vi "Cuenta.vi"(8 "error in (no error)":errorcluster, 11 "Contador Binario in":refnum<class "Contador Binario.lvclass">) -> (0 "error out":errorcluster, 3 "Contador Binario out":refnum<class "Contador Binario.lvclass">)   [LabVIEW 2020, in "Contador Binario.lvlib" / "Contador Binario.lvclass"]
uses:
  Contador Binario.lvclass
  Contador Binario.lvclass/Contador Binario.ctl
  Logging Txt/Logging Txt Messages/Save data Msg/Save data Msg.lvclass/Save data Msg.ctl
  <vilib>/ActorFramework/Message Enqueuer/Message Enqueuer.lvclass/Message Enqueuer.ctl
  <vilib>/ActorFramework/Message Enqueuer/Enqueue.vi
  Logging Txt/Logging Txt Messages/Save data Msg/Save data Msg.lvclass
  C:/Program Files (x86)/National Instruments/LabVIEW 2020/vi.lib/ActorFramework/Message/Message.lvclass
  <vilib>/ActorFramework/Message Priority Queue/Priority Enqueue.vi
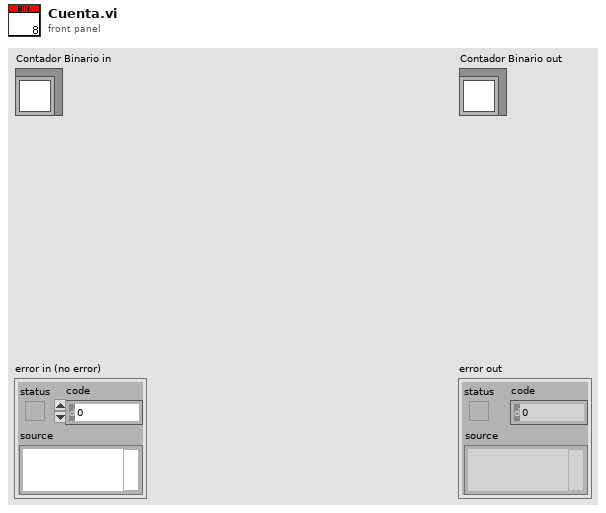
[diagram p1: front panel]
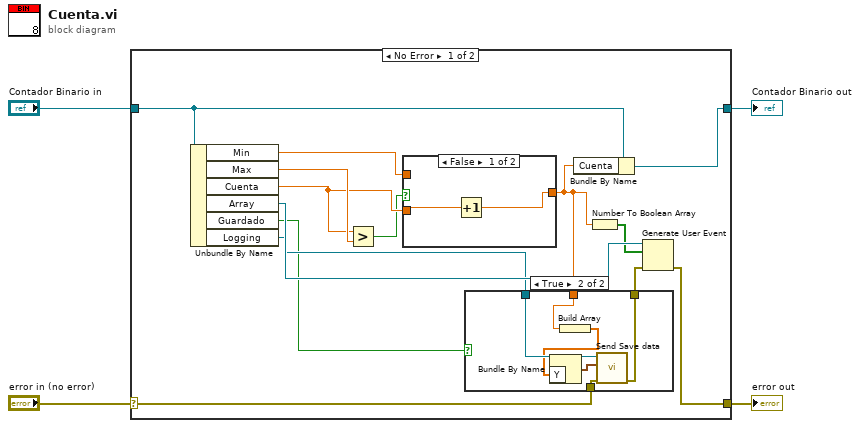
[diagram p0: block diagram]
diagram:
  n1 = case shown="No Error" "error in (no error)" {
    selector: "error in (no error)" -> [w7 w30]
    tunnel: [w5 w30] -> w3
    tunnel: [w17 w29] -> w1
    tunnel: "Contador Binario in" -> [w18 w29]
    frame No Error {
      n2 = Unbundle By Name(w18) -> ("Min"=w14:dbl, "Max"=w16:dbl, "Cuenta"=w15:dbl, "Array"=w12:refnum<user-event>, "Guardado"=w9:bool, "Logging"=w10:refnum<class "Message Enqueuer.lvclass">)
      n3 = Greater?(x=w15, y=w16) -> (0:w13:bool)
      n4 = case shown="False" w13 {
        tunnel: w15 -> [w26 _]
        tunnel: [w27 w28] -> w8
        tunnel: w14 -> [_ w28]
        frame False {
          n5 = Increment(x=w26) -> (x+1=w27:dbl)
        }
        frame True {
        }
      }
      n6 = case shown="True" w9 {
        tunnel: w10 -> [_ w25]
        tunnel: w8 -> [_ w23]
        tunnel: w7 -> [w19 w21]
        tunnel: [w19 w20] -> w6
        frame False {
        }
        frame True {
          n7 = Build Array(w23) -> (w22:dbl[])
          n8 = Bundle By Name("Y"=w22) -> (w24:waveform(dbl))  [unwired: 1 in]
          n9 = call "Send Save data.vi"("error in (no error)"=w21, "signal out"=w24, "Message Enqueuer"=w25) -> ("error out"=w20:errorcluster)  [unwired: 7 in, 1 out]
        }
      }
      n10 = Bundle By Name(cluster=w18, "Cuenta"=w8) -> (w17:refnum<class "Contador Binario.lvclass">)
      n11 = Number To Boolean Array(number=w8) -> (Boolean array=w11:bool[])
      n12 = Generate User Event(user event=w12, event data cluster=w11, error in=w6) -> (error out=w5:errorcluster)  [unwired: 1 in, 1 out]
    }
    frame Error {
    }
  }
  "error out" <- w3
  "Contador Binario out" <- w1
